vi "MTMount_logEvent_elevationInPosition.vi"(8 "error in (no error)":errorcluster, 11 "logevent_elevationInPosition_Ctl":T1) -> (0 "error out":errorcluster, 2 "function return":i32, 3 "logevent_elevationInPosition_Ctl out":T1)   [LabVIEW 2018, in "SALLV_MTMount.lvlib"]
doc: "int MTMount_shm_logEvent_elevationInPositionLV(MTMount_logevent_elevationInPositionLV *logevent_elevationInPosition_Ctl );"
uses:
  DataTypes/logevent_elevationInPosition.ctl
  SALLV_MTMount.lvlib
  SALLV_MTMount.so
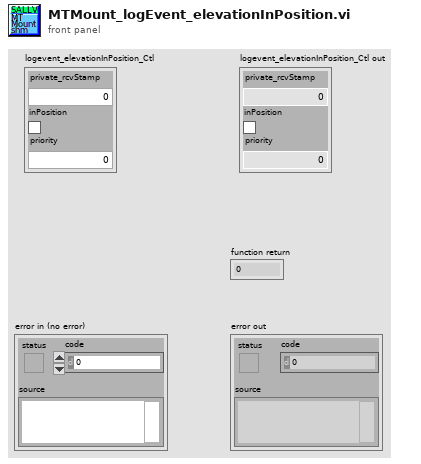
[diagram p1: front panel]
types:
  T1 = typedef "SALLV_MTMount.lvlib/logevent_elevationInPosition.ctl" = cluster{"private_rcvStamp":dbl, "inPosition":bool, "priority":i32}
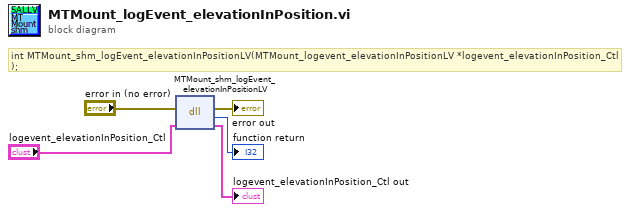
[diagram p0: block diagram]
diagram:
  # "int MTMount_shm_logEvent_elevationInPositionLV(MTMount_logevent_elevationInPositionLV *logevent_elevationInPosition_Ctl );"
  n1 = dll-call lib="home/ttsai/Documents/salLabviewApi/SALLV_MTMount/SALLV_MTMount.*" fn="MTMount_shm_logEvent_elevationInPositionLV"(error in="error in (no error)", "logevent_elevationInPosition_Ctl"="logevent_elevationInPosition_Ctl") -> (error out=→"error out":errorcluster, →"function return":i32, "logevent_elevationInPosition_Ctl"=→"logevent_elevationInPosition_Ctl out":T1)  [unwired: 2 in, 1 out]
